vi "Basic Scalar Write-Read.vi"() -> ()   [LabVIEW 2013]
uses:
  Classes/Shared Memory/Public/Controls/file mode.ctl
  Pointer Operations/Write Scalar DBL.vi
  Pointer Operations/Read Scalar DBL.vi
  Classes/Shared Memory/Shared Memory.lvclass
  Shared Memory.lvlib
panel:
  in  "write":dbl
  out "read":dbl
  in  "stop":bool
  in  "shared memory name":string="/example"
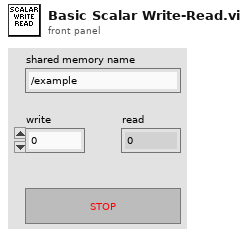
[diagram p1: front panel]
types:
  T1 = typedef "Shared Memory.lvlib/Shared Memory.lvclass/file mode.ctl" = enum16{"open", "create/replace"}
  T2 = typedef "Shared Memory.lvlib/Shared Memory.lvclass/reference.ctl" = refnum<data-value>
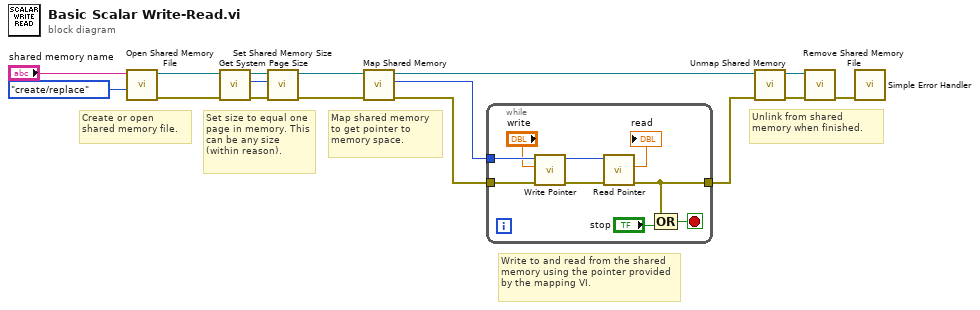
[diagram p0: block diagram]
diagram:
  # "Create or open shared memory file."
  # "Unlink from shared memory when finished."
  # "Map shared memory to get pointer to memory space."
  # "Write to and read from the shared memory using the pointer provided by the mapping VI."
  # "Set size to equal one page in memory. This can be any size (within reason)."
  n1 = call "Open Shared Memory File.vi"("file mode (open)"=file_mode."create/replace" ("file mode (default: open)"), "shared memory name"="shared memory name") -> ("error out"=w13:errorcluster, "shared memory out"=w14:T2)  [unwired: 8 in]
  n2 = call "Get System Page Size.vi"("error in (no error)"=w13, "shared memory in"=w14) -> ("error out"=w11:errorcluster, "page size (bytes)"=w10:u32, "shared memory out"=w12:T2)  [unwired: 7 in]
  n3 = call "Set Shared Memory Size.vi"("error in (no error)"=w11, "size (bytes)"=w10, "shared memory in"=w12) -> ("error out"=w9:errorcluster, "shared memory out"=w8:T2)  [unwired: 7 in]
  n4 = call "Map Shared Memory.vi"("error in (no error)"=w9, "shared memory in"=w8) -> ("error out"=w7:errorcluster, "pointer to shared memory"=w6:u64, "shared memory out"=w5:T2)  [unwired: 7 in]
  n5 = while {
    tunnel: w7 -> [w23]
    tunnel: [w18] -> w4
    tunnel: w6 -> [w22]
    stop <- w24 stop-if-true
    n6 = call-poly "Write Pointer.vi"("error in (no error)"=w23, "value"="write", "pointer in"=w22) -> ("error out"=w19:errorcluster, "pointer out"=w20:u64)  [unwired: 7 in]
    n7 = call-poly "Read Pointer.vi"("error in (no error)"=w19, "pointer in"=w20) -> ("error out"=w18:errorcluster, "value"=→"read":dbl)  [unwired: 7 in, 1 out]
    n8 = Compound Arithmetic op=OR(w18, "stop") -> (w24:bool)
  }
  n9 = call "Unmap Shared Memory.vi"("error in (no error)"=w4, "shared memory in"=w5) -> ("error out"=w3:errorcluster, "shared memory out"=w2:T2)  [unwired: 8 in]
  n10 = call "Remove Shared Memory File.vi"("error in (no error)"=w3, "shared memory in"=w2) -> ("error out"=w1:errorcluster)  [unwired: 8 in, 1 out]
  n11 = call <vilib>:"Simple Error Handler.vi"("error in (no error)"=w1) -> ()  [unwired: 4 in, 5 out]
